vi "Update Energized.vi"(6 "Time":dbl, 8 "error in (no error)":errorcluster, 11 "2WayValve in":refnum<class "2WayValveH.lvclass">) -> (0 "error out":errorcluster, 3 "2WayValve out":refnum<class "2WayValveH.lvclass">)   [LabVIEW 2020, in "VolatusGUIElements.lvlib" / "2WayValveH.lvclass"]
uses:
  2WayValveH.lvclass
  2WayValveH.lvclass/2WayValveH.ctl
  lv-vecto/Vecto/Channel/Channel.lvclass/Channel.ctl
  lv-vecto/Vecto/Group/Value by Index.vi
  lv-vecto/Vecto/Channel/Channel.lvclass
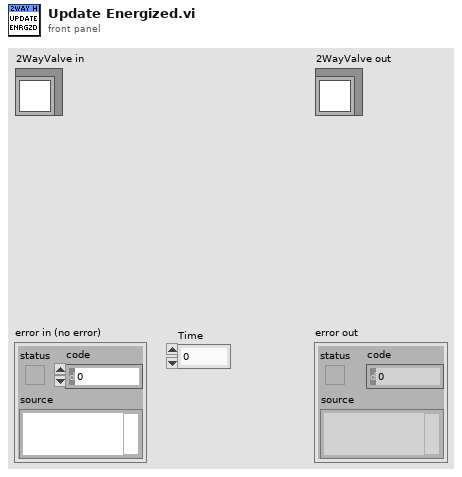
[diagram p1: front panel]
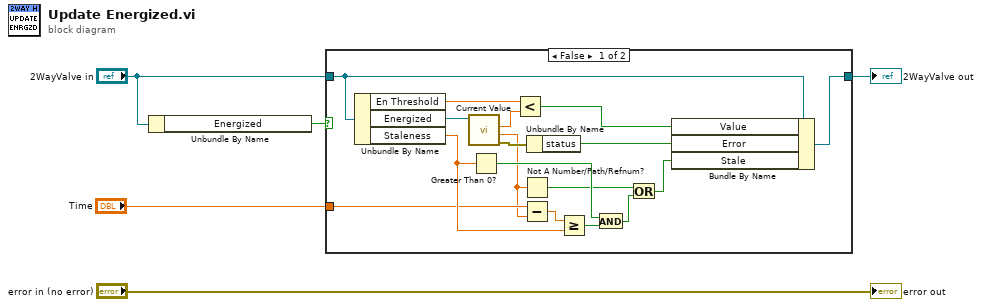
[diagram p0: block diagram]
diagram:
  n1 = Unbundle By Name("2WayValve in") -> ("Energized"=w2:bool)
  n2 = case shown="False" w2 {
    tunnel: [w9 w23] -> w4
    tunnel: "2WayValve in" -> [w10 w23]
    tunnel: "Time" -> [w15 _]
    frame False {
      n3 = Unbundle By Name(w10) -> ("En Threshold"=w8:dbl, "Energized"=w21:refnum<class "Channel.lvclass">, "Staleness"=w18:dbl)
      n4 = call "Current Value.vi"("Channel in"=w21) -> ("error out"=w22:errorcluster, "Timestamp"=w14:dbl, "Scaled"=w7:dbl)  [unwired: 6 in, 2 out]
      n5 = Greater Than 0?(x=w18) -> (x > 0?=w16:bool)
      n6 = Less?(x=w8, y=w7) -> (x < y?=w6:bool)
      n7 = Not A Number/Path/Refnum?(number/path/refnum=w14) -> (NaN/Path/Refnum?=w13:bool)
      n8 = Subtract(x=w15, y=w14) -> (x-y=w20:dbl)
      n9 = Unbundle By Name(w22) -> ("status"=w19:bool)
      n10 = Greater Or Equal?(x=w20, y=w18) -> (x >= y?=w17:bool)
      n11 = And(x=w16, y=w17) -> (x .and. y?=w12:bool)
      n12 = Or(x=w13, y=w12) -> (x .or. y?=w11:bool)
      n13 = Bundle By Name(cluster=w10, "Value"=w6, "Error"=w19, "Stale"=w11) -> (w9:refnum<class "2WayValveH.lvclass">)
    }
    frame True {
      # "Energized Unused"
    }
  }
  "2WayValve out" <- w4
  "error out" <- "error in (no error)"
